vi "4461 - Create AO waveforms.vi"(6 "time delay":dbl, 8 "error in (no error)":errorcluster, 9 "sampling info":cluster{"Fs":dbl, "#s":dbl}={"Fs"=1000.0, "#s"=1000.0} {"Fs" format="%.2p"}, 10 "reset signal":bool, 11 "AO":T1={"AO amp (V)"=[0.1, 0.09, 0.08, 0.07, 0.06, 0.05, 0.04, 0.03], "AO DC (V)"=[0.0, 0.0, 0.0, 0.0, 0.0, 0.0, 0.0, 0.0], "AO f (Hz)"=[13.0, 13.0, 13.0, 13.0, 13.0, 13.0, 13.0, 13.0], "AO phi (deg)"=[0.0, 0.0, 0.0, 0.0, 0.0, 0.0, 0.0, 0.0], "function"=[enum."Sine Wave", enum."Sine Wave", enum."Sine Wave", enum."Sine Wave", enum."Sine Wave", enum."Sine Wave", enum."Sine Wave", enum."Sine Wave"]} {"AO DC (V)" format="%#_6p"; "AO amp (V)" format="%#_6p"}) -> (0 "error out":errorcluster, 1 "phase out":dbl[](array[numeric]), 2 "AO Array":waveform(dbl)[](array[waveform]), 3 "AO 2":T1={"AO amp (V)"=[0.1, 0.09, 0.08, 0.07, 0.06, 0.05, 0.04, 0.03], "AO DC (V)"=[0.0, 0.0, 0.0, 0.0, 0.0, 0.0, 0.0, 0.0], "AO f (Hz)"=[13.0, 13.0, 13.0, 13.0, 13.0, 13.0, 13.0, 13.0], "AO phi (deg)"=[0.0, 0.0, 0.0, 0.0, 0.0, 0.0, 0.0, 0.0], "function"=[enum."Sine Wave", enum."Sine Wave", enum."Sine Wave", enum."Sine Wave", enum."Sine Wave", enum."Sine Wave", enum."Sine Wave", enum."Sine Wave"]} {"AO DC (V)" format="%#_6p"; "AO amp (V)" format="%#_6p"})   [LabVIEW 2016]
uses:
  <vilib>/Analysis/2dsp.llb/Decimate (single shot).vi
  <vilib>/Analysis/2dsp.llb/Decimate (single shot, DBL).vi
  <vilib>/Utility/error.llb/Error Cluster From Error Code.vi
  <vilib>/measure/NI_MABase.lvlib
panel:
  out "Waveform Chart":dbl[][](graph)
  out "Waveform Graph 2":waveform(dbl)[](graph)
  out "Numeric":i32
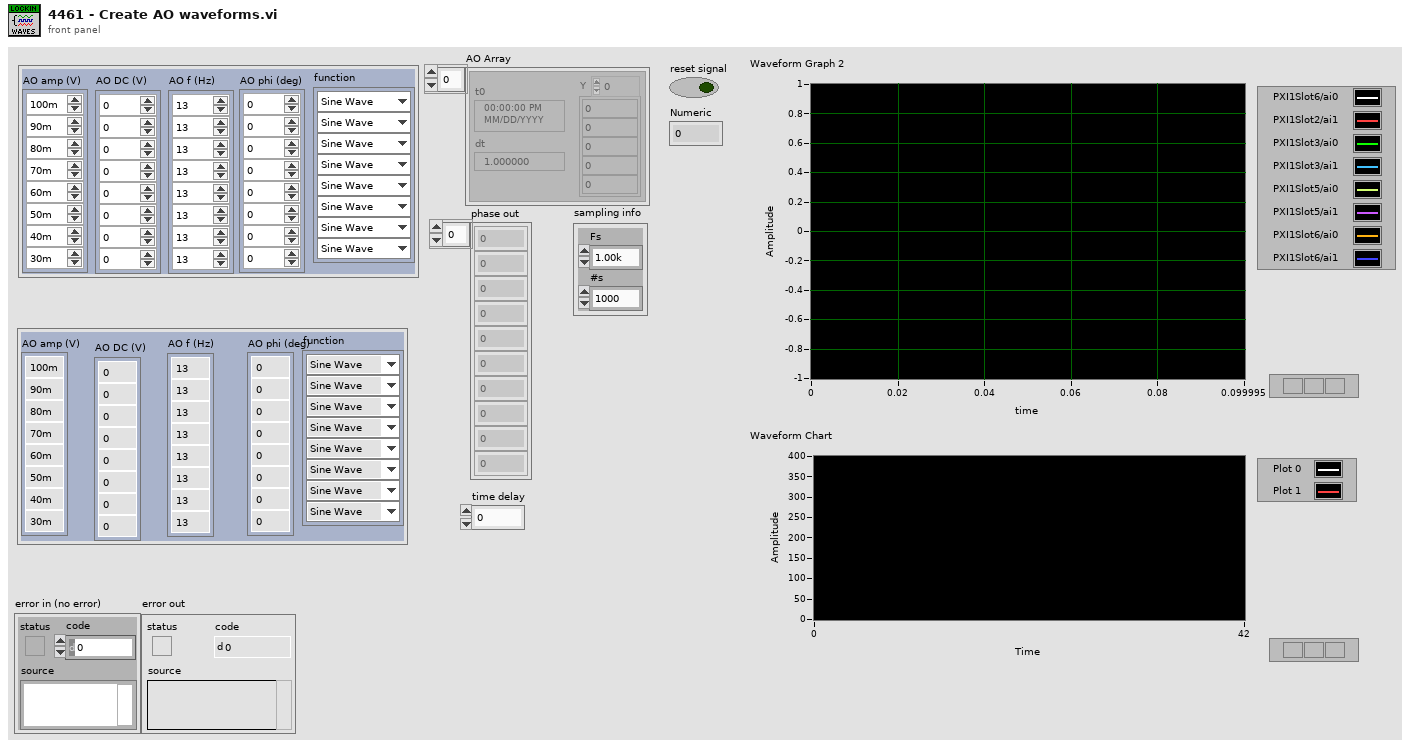
[diagram p1: front panel]
types:
  T1 = cluster{"AO amp (V)":dbl[], "AO DC (V)":dbl[], "AO f (Hz)":dbl[], "AO phi (deg)":dbl[], "function":enum16{"Sine Wave", "Triangle Wave", "Square Wave", "Sawtooth Wave"}[]}
  T2 = enum16{"Sine Wave", "Triangle Wave", "Square Wave", "Sawtooth Wave"}[]
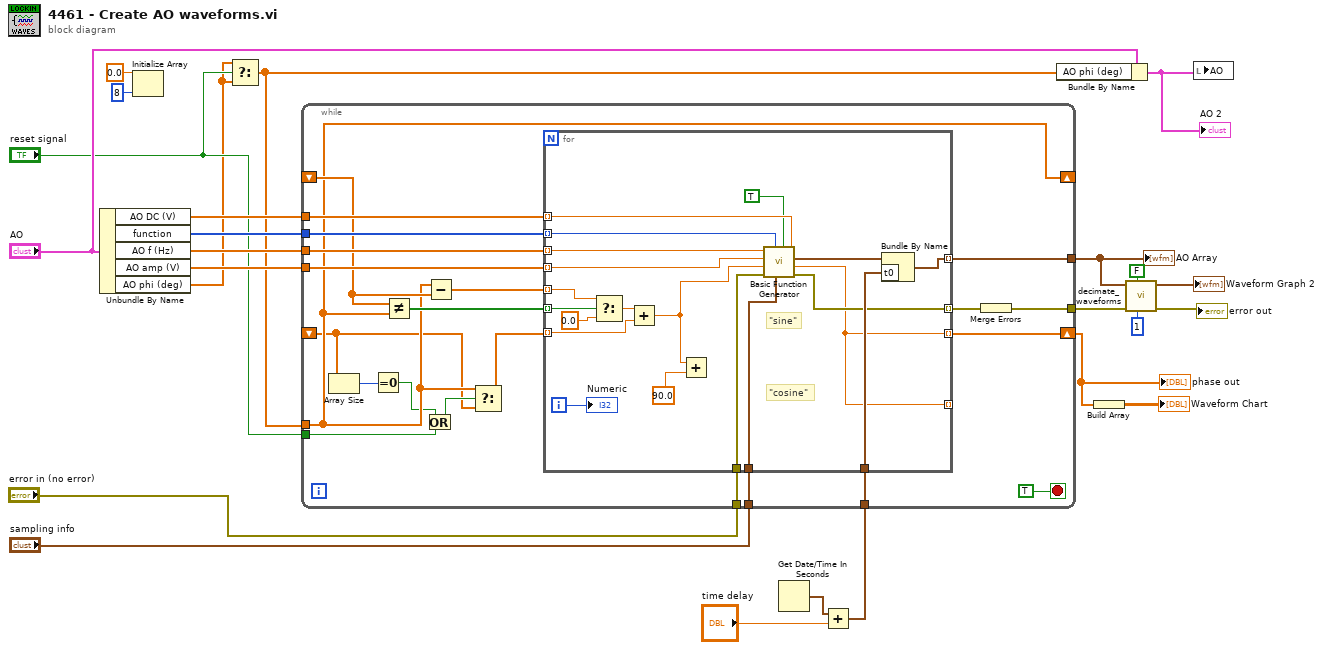
[diagram p0: block diagram]
diagram:
  n1 = Unbundle By Name("AO") -> ("AO DC (V)"=w23:dbl[], "function"=w24:T2, "AO f (Hz)"=w20:dbl[], "AO amp (V)"=w21:dbl[], "AO phi (deg)"=w1:dbl[])
  n2 = Initialize Array(0.0 ("element"), 8 ("dimension size")) -> ()  [unwired: 1 out]
  n3 = Select(t=w1, s="reset signal", f=w1) -> (s? t:f=w15:dbl[])
  n4 = Get Date/Time In Seconds() -> (seconds since 1Jan1904=w6:timestamp)
  n5 = Add(x=w6, y="time delay") -> (x+y=w4:timestamp)
  n6 = while {
    tunnel: w24 -> [w46]
    tunnel: w23 -> [w45]
    tunnel: "sampling info" -> [w44]
    tunnel: [w43] -> w11
    tunnel: w21 -> [w42]
    tunnel: w15 -> [w33]
    tunnel: w20 -> [w41]
    shift-right: [w33] -> _
    shift-left: _ -> [w38]
    shift-right: [w36] -> w2
    shift-left: _ -> [w25]
    tunnel: w4 -> [w35]
    tunnel: "reset signal" -> [w30]
    tunnel: "error in (no error)" -> [w28]
    tunnel: [w26] -> w8
    stop <- TRUE stop-if-true
    n7 = Array Size(array=w25) -> (size(s)=w34:i32)
    n8 = Equal To 0?(x=w34) -> (x = 0?=w31:bool)
    n9 = Not Equal?(x=w38, y=w33) -> (x != y?=w39:bool[])
    n10 = Or(x=w31, y=w30) -> (x .or. y?=w32:bool)
    n11 = Subtract(x=w33, y=w38) -> (x-y=w37:dbl[])
    n12 = Select(t=w33, s=w32, f=w25) -> (s? t:f=w29:dbl[])
    n13 = for {
      tunnel: w46 -> [w66] mode=indexing
      tunnel: w41 -> [w65] mode=indexing
      tunnel: w42 -> [w64] mode=indexing
      tunnel: w45 -> [w63] mode=indexing
      tunnel: [w52] -> w43 mode=indexing
      tunnel: w44 -> [w53]
      tunnel: w39 -> [w57] mode=indexing
      tunnel: w37 -> [w59] mode=indexing
      tunnel: [w49] -> w36 mode=indexing
      tunnel: w29 -> [w48] mode=indexing
      tunnel: w35 -> [w56]
      tunnel: [w49] -> _ mode=indexing
      tunnel: w28 -> [w51]
      tunnel: [w50] -> w27 mode=indexing
      i -> [w55]
      # "\"cosine\""
      # "\"sine\""
      n14 = Select(t=w59, s=w57, f=0.0) -> (s? t:f=w60:dbl)
      n15 = Add(x=w60, y=w48) -> (x+y=w47:dbl)
      n16 = Add(x=w47, y=90.0) -> ()  [unwired: 1 out]
      n17 = call <vilib>:"Basic Function Generator.vi"("offset"=w63, "reset signal"=TRUE, "sampling info"=w53, "signal type"=w66, "error in (no error)"=w51, "phase"=w47, "amplitude"=w64, "frequency"=w65) -> ("error out"=w50:errorcluster, "phase out"=w49:dbl, "signal out"=w62:waveform(dbl))  [unwired: 1 in]
      n18 = Bundle By Name(cluster=w62, "t0"=w56) -> (w52:waveform(dbl))
      "Numeric" <- w55
    }
    n19 = Merge Errors(w27) -> (w26:errorcluster)
  }
  "AO Array" <- w11
  "phase out" <- w2
  n20 = Bundle By Name(cluster="AO", "AO phi (deg)"=w15) -> (w16:T1)
  "AO 2" <- w16
  n21 = Build Array(w2) -> (→"Waveform Chart":dbl[][])
  n22 = call "decimate_waveforms.vi"("decimating factor"=1, "averaging"=FALSE, "error in (no error)"=w8, "Input Signal"=w11) -> ("error out"=→"error out":errorcluster, "Decimated Waveforms"=→"Waveform Graph 2":waveform(dbl)[])  [unwired: 6 in]
  n23 = local write "AO"(w16) -> ()
